vi "ZCR_test_signal_regeneration.vi"() -> ()   [LabVIEW 2020, in "Library Commun.lvlib" / "Nodon_ZCR.lvclass"]
uses:
  Nodon_ZCR.lvclass
  <vilib>/Utility/miscctls.llb/LVRangeTypeDef.ctl
  <vilib>/Analysis/baseanly.llb/Mean (DBL).vi
  <vilib>/measure/matone.llb/Extract Single Tone Information 1 Chan.vi
  Nodon_ZCR.lvclass/Nodon_ZCR.ctl
  <vilib>/measure/NI_MABase.lvlib
  <vilib>/measure/NI_MAPro.lvlib
  <vilib>/Analysis/NI_AALBase.lvlib
  <vilib>/Analysis/NI_AALPro.lvlib
  <vilib>/ptbypt/NI_PtbyPt.lvlib
panel:
  out "FINAL OFF":i32[](array[numeric])
  out "Array 3":i32[](array[numeric])
  out "FINAL ON":i32[](array[numeric])
  out "OFF ARRAY FINAL":i32[](array[numeric])
  out "ON ARRAY FINAL":i32[](array[numeric])
  in  "Coeff":dbl
  in  "Point 2":i32
  out "Delta OFF":i32[](array[numeric])
  out "OFF":i32[](array[numeric])
  out "Array":i32[](array[numeric])
  in  "Point":i32
  out "Waveform Graph 4":waveform(dbl)[](graph)
  out "Waveform Graph 3":waveform(dbl)(graph)
  in  "amplitude":dbl=1.0 format="%.2p"
  out "Waveform Graph 2":waveform(dbl)(graph)
  in  "ZCR ON":waveform(dbl)[](graph)=[{"t0"=timestamp(3707890383.8976955 s since 1904-01-01), "dt"=9.999999999999999e-05, "Y"=array[20000 elements], "attributes"=variant("NI_ChannelName"=variant(string "Tension_0"), "NI_UnitDescription"=variant(string "Volts"))}, {"t0"=timestamp(3707890383.8977456 s since 1904-01-01), "dt"=9.999999999999999e-05, "Y"=array[20000 elements], "attributes"=variant("NI_ChannelName"=variant(string "Tension_1"), "NI_UnitDescription"=variant(string "Volts"))}]
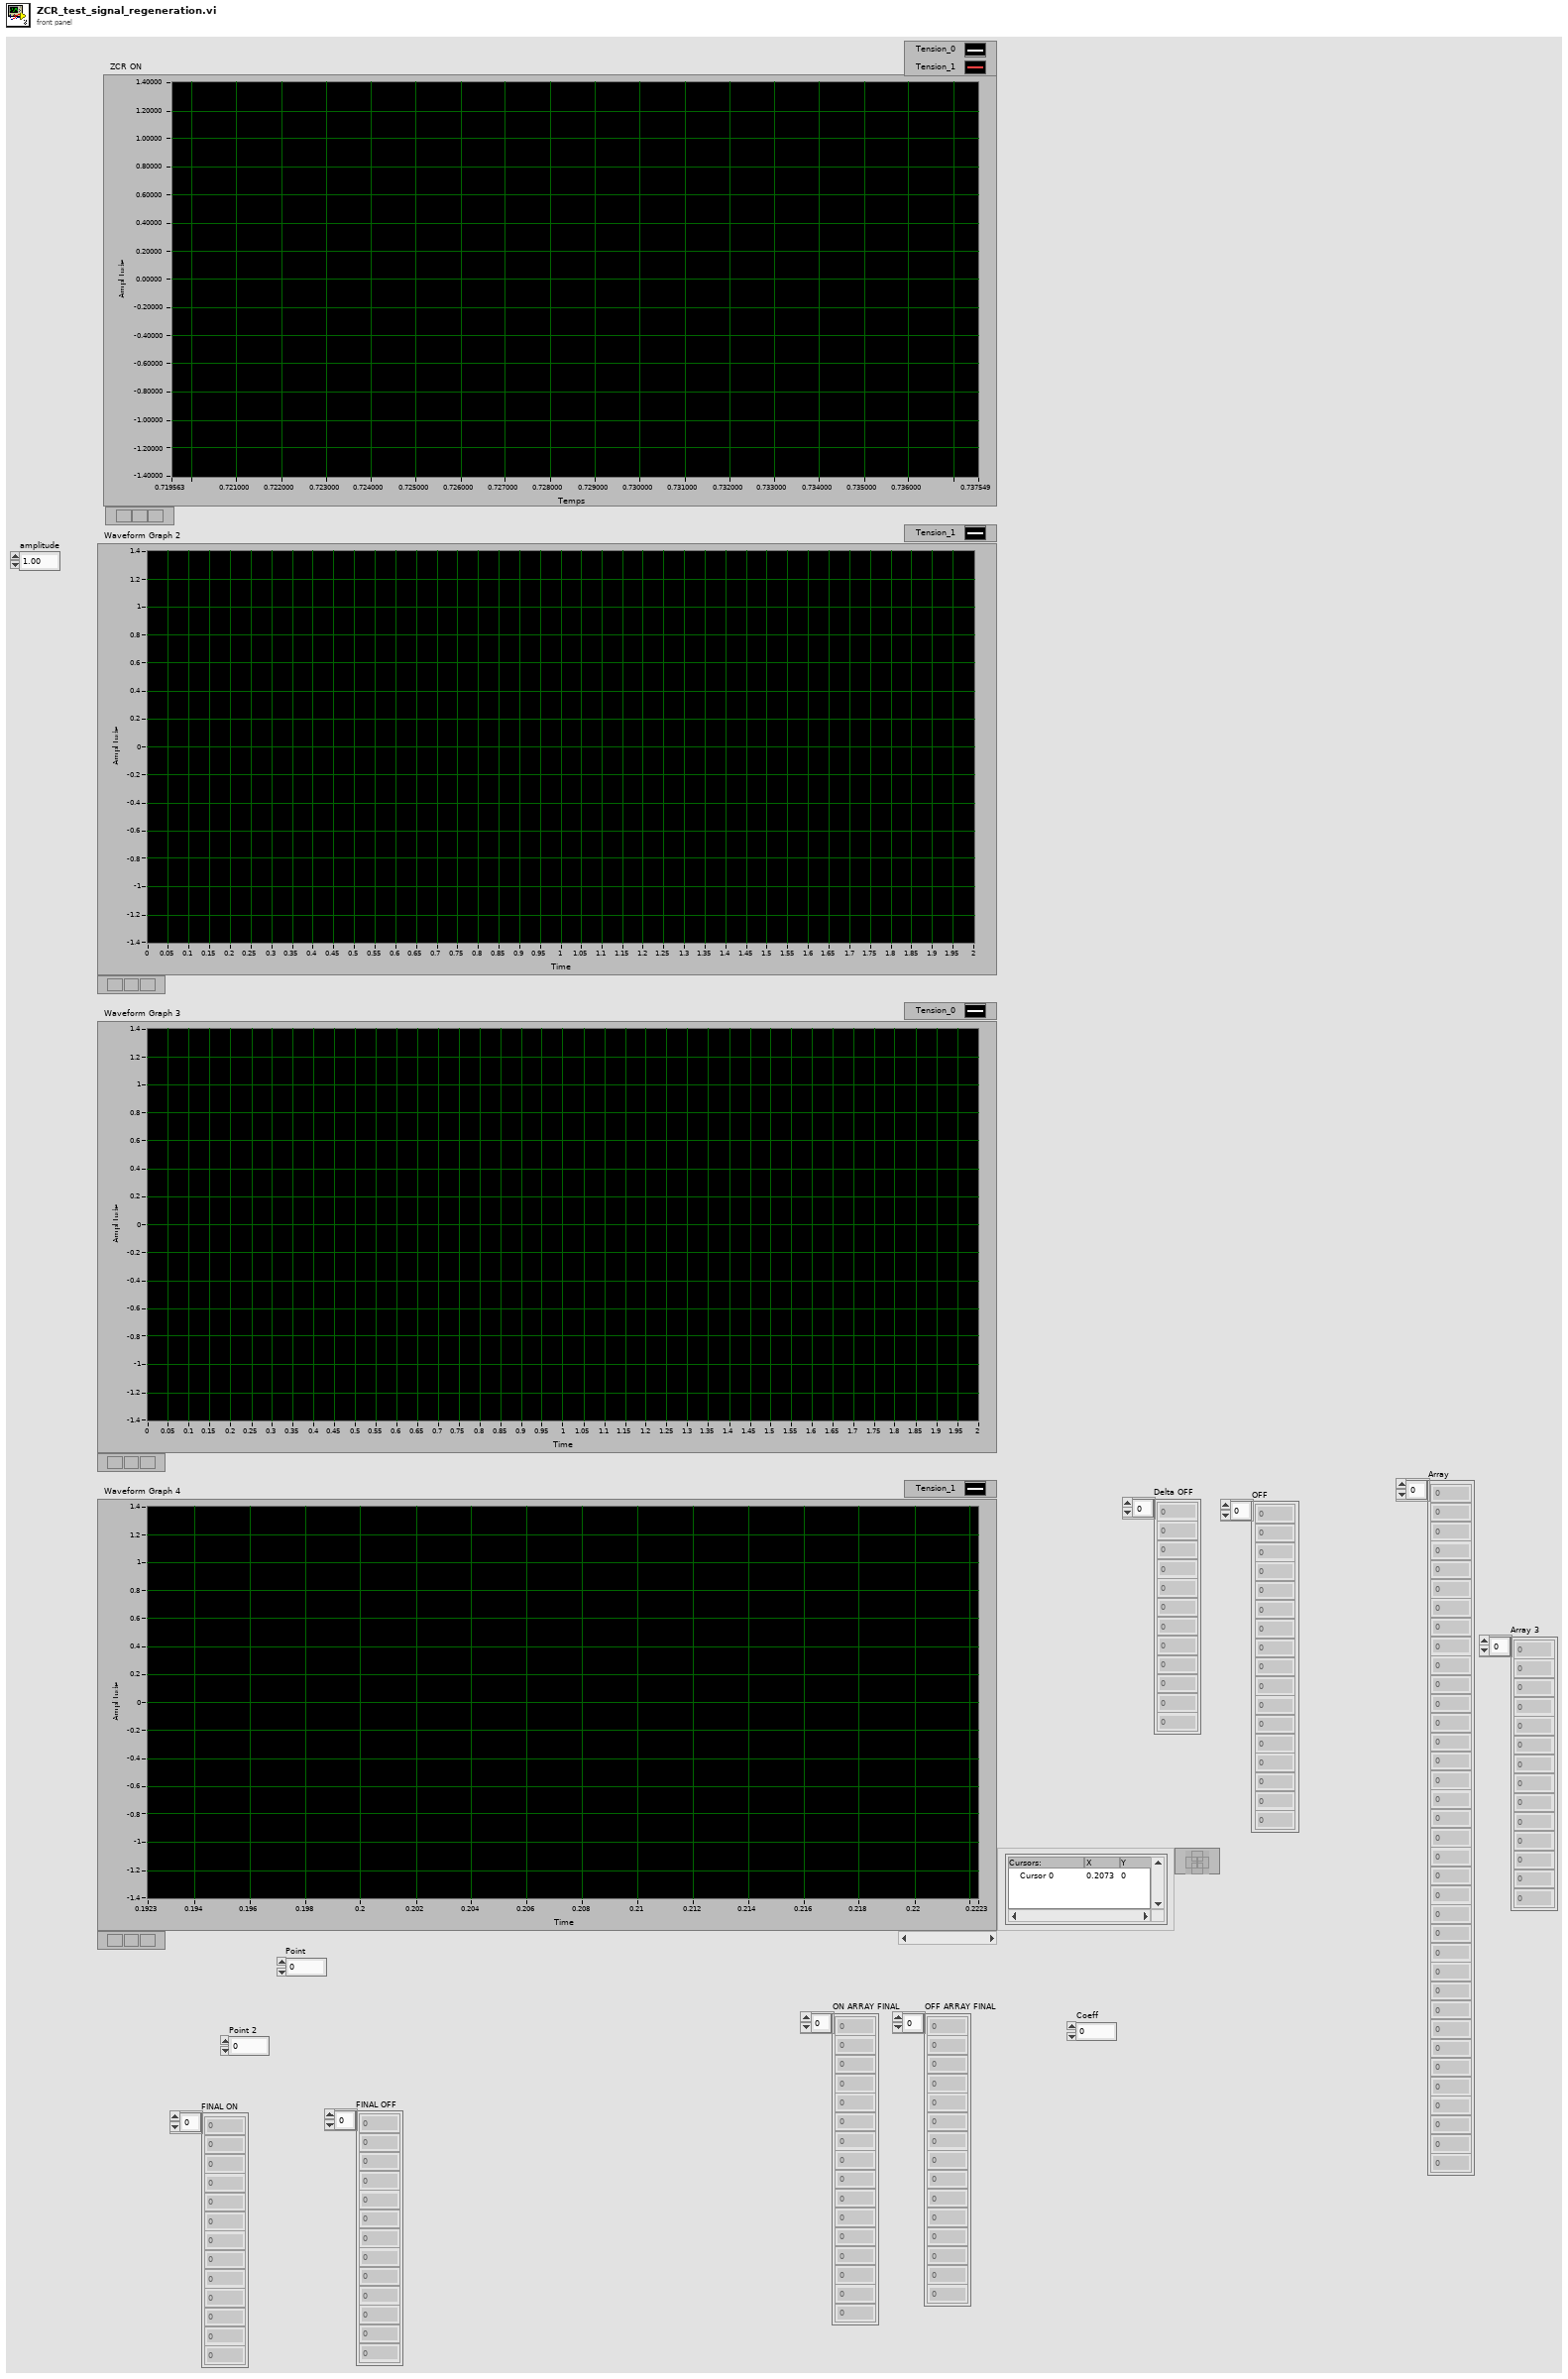
[diagram p1: front panel]
types:
  T1 = typedef "LVRangeTypeDef.ctl" = cluster{"Minimum":dbl, "Maximum":dbl, "Increment":dbl, "Minor Increment":dbl, "Start":dbl}
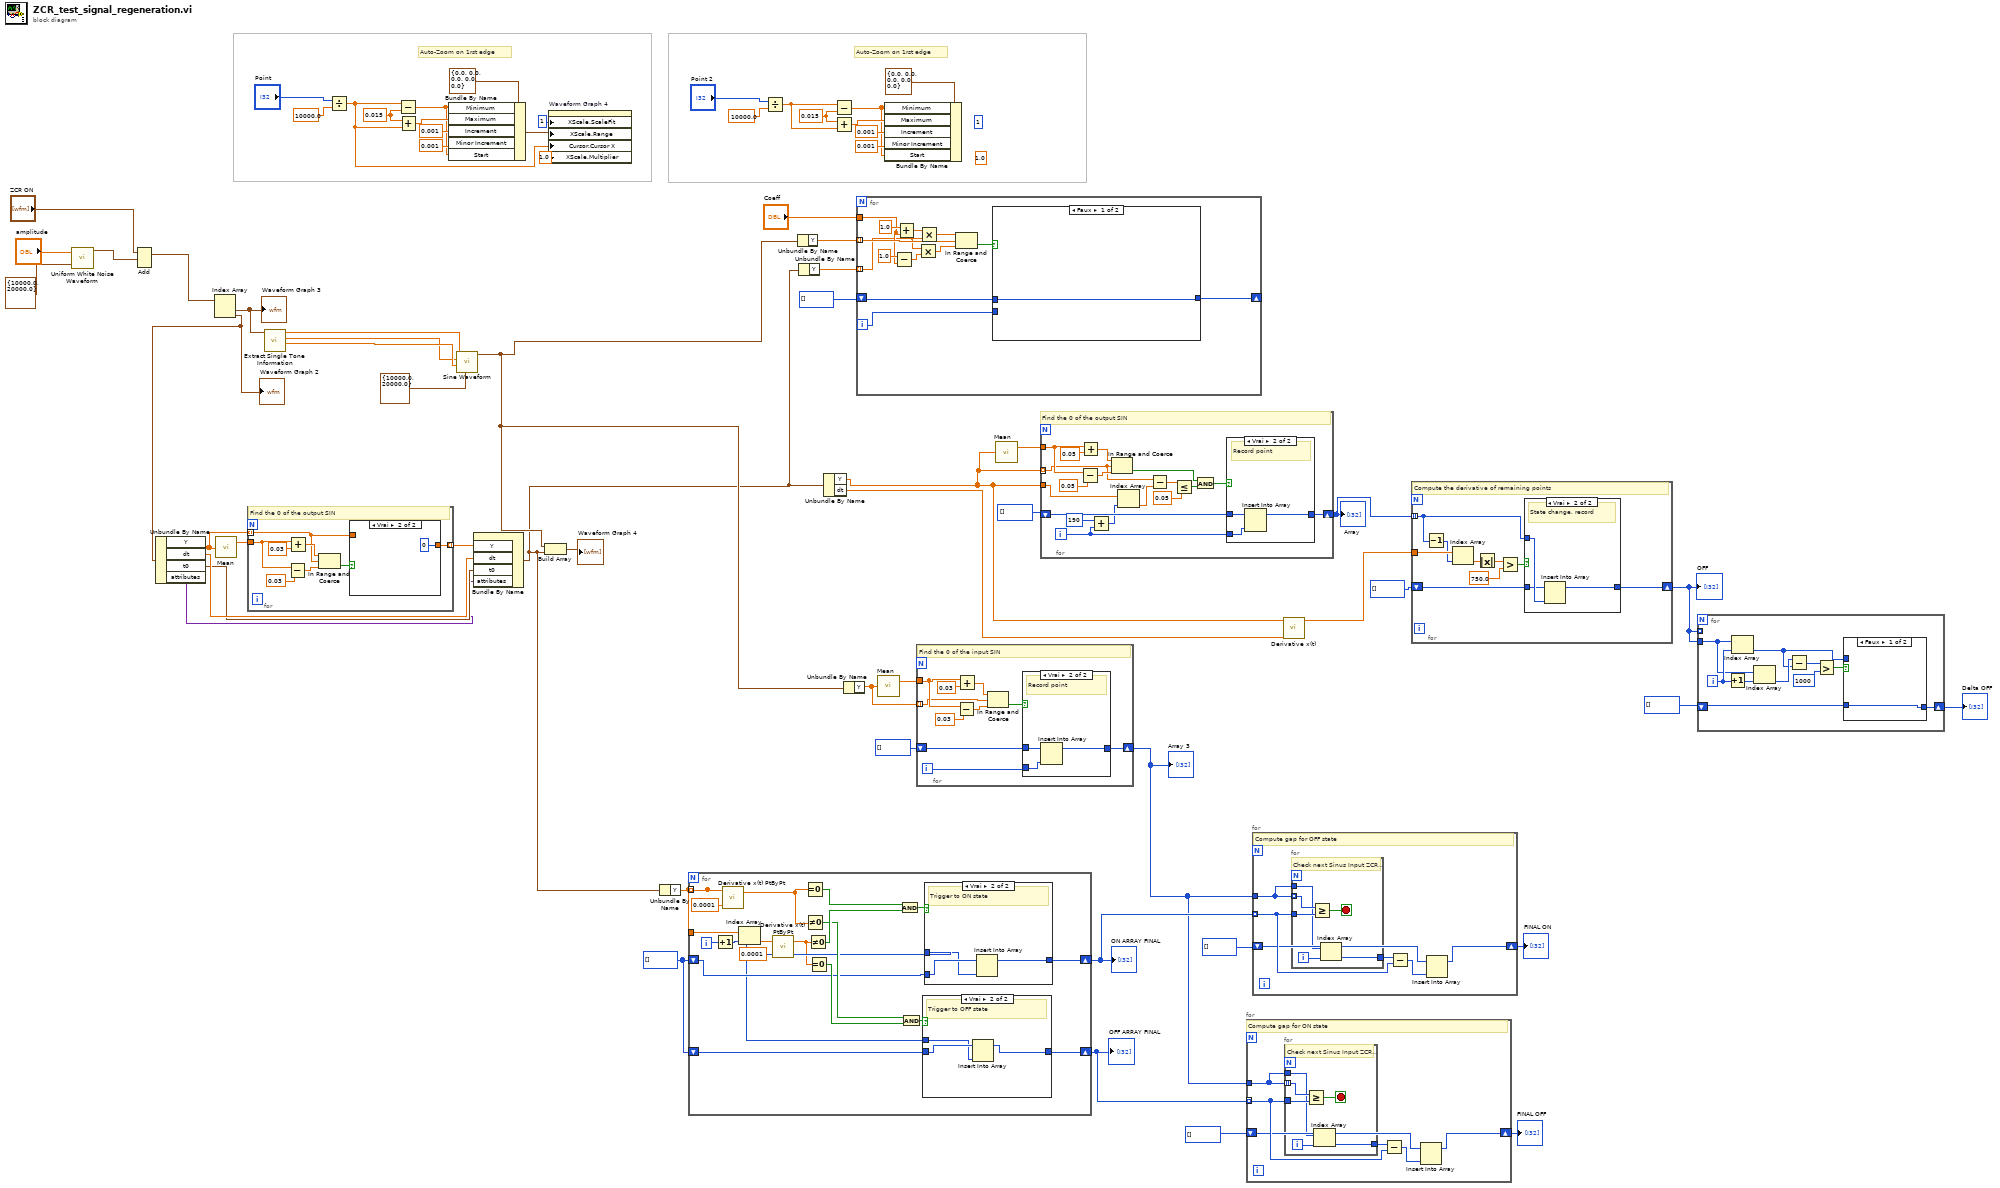
[diagram p0: block diagram]
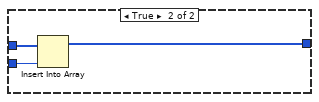
[diagram p5: hidden frame]
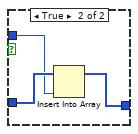
[diagram p7: hidden frame]
diagram:
  w17 = i32[] []
  (unwired) 1.0 ("X Scale.Offset and Multiplier:Multiplier")
  (unwired) u8 1 ("X Scale.Scale Fit")
  w37 = 0.015
  w60 = 0.015
  # "Auto-Zoom on 1rst edge"
  # "Auto-Zoom on 1rst edge"
  n1 = call <vilib>:"Uniform White Noise Waveform.vi"("sampling info"=cluster{"Fs":dbl, "#s":dbl} {"Fs"=10000.0, "#s"=20000.0}, "amplitude"="amplitude") -> ("signal out"=w5:waveform(dbl))  [unwired: 8 in, 1 out]
  n2 = Add(1:w5, 2:"ZCR ON") -> (0:w3:waveform(dbl)[])  [unwired: 1 in, 1 out]
  n3 = Index Array(array=w3) -> (element #1=w21:waveform(dbl), element #2=w4:waveform(dbl))  [unwired: 2 in]
  "Waveform Graph 2" <- w4
  "Waveform Graph 3" <- w21
  n4 = Unbundle By Name(w4) -> ("Y"=w24:dbl[], "dt"=w27:dbl, "t0"=w26:timestamp, "attributes"=w25:variant)
  n5 = call-poly <vilib>:"Mean.vi"("X"=w24) -> ("mean"=w29:dbl)  [unwired: 1 out]
  n6 = for {
    tunnel: w29 -> [w71]
    tunnel: [w69] -> w28 mode=indexing
    tunnel: w24 -> [w68] mode=indexing
    # "Find the 0 of the output SIN"
    n7 = Subtract(x=w71, y=0.03) -> (x-y=w73:dbl)
    n8 = Add(x=w71, y=0.03) -> (x+y=w75:dbl)
    n9 = In Range and Coerce(upper limit=w75, x=w68, lower limit=w73) -> (In Range?=w70:bool)  [unwired: 1 out]
    n10 = case shown="Vrai" w70 {
      tunnel: w68 -> [w76 _]
      tunnel: [w76 0] -> w69
      frame False {
      }
      frame True {
      }
    }
  }
  n11 = call-poly <vilib>:"Extract Single Tone Information.vi"("time signal in"=w21) -> ("detected phase (deg)"=w64:dbl, "detected amplitude"=w63:dbl, "detected frequency"=w62:dbl)  [unwired: 5 in, 3 out]
  n12 = Divide(x="Point", y=10000.0) -> (x/y=w51:dbl)
  n13 = Subtract(x=w51, y=w60) -> (x-y=w55:dbl)
  n14 = Add(x=w60, y=w51) -> (x+y=w58:dbl)
  n15 = Bundle By Name(cluster=T1 {"Minimum"=0.0, "Maximum"=0.0, "Increment"=0.0, "Minor Increment"=0.0, "Start"=0.0} ("X Scale.Range"), "Minimum"=w55, "Maximum"=w58, "Increment"=0.001, "Minor Increment"=0.001, "Start"=w55) -> (w54:T1)
  n16 = call <vilib>:"Sine Waveform.vi"("sampling info"=cluster{"Fs":dbl, "#s":dbl} {"Fs"=10000.0, "#s"=20000.0}, "phase"=w64, "amplitude"=w63, "frequency"=w62) -> ("signal out"=w2:waveform(dbl))  [unwired: 6 in, 1 out]
  n17 = Bundle By Name("Y"=w28, "dt"=w27, "t0"=w26, "attributes"=w25) -> (w1:waveform(dbl))  [unwired: 1 in]
  n18 = Build Array(w2, w1) -> (→"Waveform Graph 4":waveform(dbl)[])
  n19 = property on="Waveform Graph 4" class="GraphWF (strict)"("XScale.ScaleFit"=u8 1 ("X Scale.Scale Fit"), "XScale.Range"=w54, "Cursor.Cursor X"=w51, "XScale.Multiplier"=1.0 ("X Scale.Offset and Multiplier:Multiplier")) -> ()  [unwired: 2 in, 2 out]
  n20 = Unbundle By Name(w1) -> ("Y"=w18:dbl[])
  n21 = for {
    tunnel: [w83] -> _ mode=indexing
    tunnel: w18 -> [w83] mode=indexing
    tunnel: w18 -> [w96]
    shift-right: [w85] -> w11
    shift-left: w17 -> [w88]
    shift-right: [w84] -> w9
    shift-left: w17 -> [w87]
    i -> [w86]
    n22 = Increment(x=w86) -> (x+1=w95:i32)
    n23 = call <vilib>:"Derivative x(t) PtByPt.vi"("dt"=0.0001, "x"=w83) -> ("dx/dt"=w82:dbl)  [unwired: 2 in, 1 out]
    n24 = Index Array(array=w96, index=w95) -> (element=w80:dbl)
    n25 = call <vilib>:"Derivative x(t) PtByPt.vi"("dt"=0.0001, "x"=w80) -> ("dx/dt"=w79:dbl)  [unwired: 2 in, 1 out]
    n26 = Equal To 0?(x=w82) -> (x = 0?=w93:bool)
    n27 = Not Equal To 0?(x=w82) -> (x != 0?=w90:bool)
    n28 = Not Equal To 0?(x=w79) -> (x != 0?=w94:bool)
    n29 = Equal To 0?(x=w79) -> (x = 0?=w91:bool)
    n30 = And(x=w93, y=w94) -> (x .and. y?=w92:bool)
    n31 = And(x=w90, y=w91) -> (x .and. y?=w89:bool)
    n32 = case shown="Vrai" w89 {
      tunnel: w87 -> [w97 w100]
      tunnel: w86 -> [_ w99]
      tunnel: [w97 w98] -> w84
      frame False {
      }
      frame True {
        # "Trigger to OFF state"
        n33 = Insert Into Array(array=w100, new element=w99) -> (w98:i32[])  [unwired: 1 in]
      }
    }
    n34 = case shown="Vrai" w92 {
      tunnel: w88 -> [w101 w104]
      tunnel: w86 -> [_ w103]
      tunnel: [w101 w102] -> w85
      frame False {
      }
      frame True {
        # "Trigger to ON state"
        n35 = Insert Into Array(array=w104, new element=w103) -> (w102:i32[])  [unwired: 1 in]
      }
    }
  }
  "ON ARRAY FINAL" <- w11
  "OFF ARRAY FINAL" <- w9
  n36 = Divide(x="Point 2", y=10000.0) -> (x/y=w31:dbl)
  n37 = Unbundle By Name(w2) -> ("Y"=w23:dbl[])
  n38 = Unbundle By Name(w1) -> ("Y"=w22:dbl[])
  n39 = Unbundle By Name(w1) -> ("Y"=w45:dbl[], "dt"=w44:dbl)
  n40 = Subtract(x=w31, y=w37) -> (x-y=w32:dbl)
  n41 = Add(x=w37, y=w31) -> (x+y=w35:dbl)
  n42 = Unbundle By Name(w2) -> ("Y"=w14:dbl[])
  n43 = for {
    tunnel: w23 -> [w117] mode=indexing
    tunnel: w22 -> [w110] mode=indexing
    tunnel: "Coeff" -> [w114]
    shift-right: [w105] -> _
    shift-left: i32[] [] -> [w107]
    i -> [w106]
    n44 = Subtract(x=1.0, y=w114) -> (x-y=w111:dbl)
    n45 = Add(x=1.0, y=w114) -> (x+y=w113:dbl)
    n46 = Multiply(x=w110, y=w111) -> (x*y=w109:dbl)
    n47 = Multiply(x=w113, y=w110) -> (x*y=w112:dbl)
    n48 = In Range and Coerce(upper limit=w112, x=w117, lower limit=w109) -> (In Range?=w108:bool)  [unwired: 1 out]
    n49 = case shown="Faux" w108 {
      tunnel: w107 -> [w118 w121]
      tunnel: w106 -> [_ w120]
      tunnel: [w118 w119] -> w105
      frame False {
      }
      frame True {
        n50 = Insert Into Array(array=w121, new element=w120) -> (w119:i32[])  [unwired: 1 in]
      }
    }
  }
  n51 = call-poly <vilib>:"Mean.vi"("X"=w14) -> ("mean"=w16:dbl)  [unwired: 1 out]
  n52 = Bundle By Name(cluster=T1 {"Minimum"=0.0, "Maximum"=0.0, "Increment"=0.0, "Minor Increment"=0.0, "Start"=0.0} ("X Scale.Range"), "Minimum"=w32, "Maximum"=w35, "Increment"=0.001, "Minor Increment"=0.001, "Start"=w32) -> ()  [unwired: 1 out]
  n53 = for {
    tunnel: w14 -> [w126] mode=indexing
    tunnel: w16 -> [w127]
    shift-right: [w122] -> w10
    shift-left: i32[] [] -> [w123]
    i -> [w124]
    # "Find the 0 of the input SIN"
    n54 = Subtract(x=w127, y=0.03) -> (x-y=w129:dbl)
    n55 = Add(x=w127, y=0.03) -> (x+y=w131:dbl)
    n56 = In Range and Coerce(upper limit=w131, x=w126, lower limit=w129) -> (In Range?=w125:bool)  [unwired: 1 out]
    n57 = case shown="Vrai" w125 {
      tunnel: w124 -> [_ w135]
      tunnel: w123 -> [w132 w134]
      tunnel: [w132 w133] -> w122
      frame False {
        # "do nothing"
      }
      frame True {
        # "Record point"
        n58 = Insert Into Array(array=w134, new element=w135) -> (w133:i32[])  [unwired: 1 in]
      }
    }
  }
  "Array 3" <- w10
  n59 = call-poly <vilib>:"Mean.vi"("X"=w45) -> ("mean"=w48:dbl)  [unwired: 1 out]
  n60 = for {
    tunnel: w45 -> [w145] mode=indexing
    tunnel: w48 -> [w149]
    shift-right: [w147] -> w46
    shift-left: i32[] [] -> [w148]
    tunnel: w45 -> [w146]
    i -> [w137]
    # "Find the 0 of the output SIN"
    n61 = Subtract(x=w149, y=0.05) -> (x-y=w151:dbl)
    n62 = Add(x=w149, y=0.05) -> (x+y=w153:dbl)
    n63 = Add(x=190, y=w137) -> (x+y=w138:i32)
    n64 = In Range and Coerce(upper limit=w153, x=w145, lower limit=w151) -> (In Range?=w140:bool)  [unwired: 1 out]
    n65 = Index Array(array=w146, index=w138) -> (element=w144:dbl)
    n66 = Subtract(x=w145, y=w144) -> (x-y=w143:dbl)
    n67 = Less Or Equal?(x=w143, y=0.05) -> (x <= y?=w141:bool)
    n68 = And(x=w140, y=w141) -> (x .and. y?=w139:bool)
    n69 = case shown="Vrai" w139 {
      tunnel: w137 -> [_ w157]
      tunnel: w148 -> [w154 w156]
      tunnel: [w154 w155] -> w147
      frame False {
        # "do nothing"
      }
      frame True {
        # "Record point"
        n70 = Insert Into Array(array=w156, new element=w157) -> (w155:i32[])  [unwired: 1 in]
      }
    }
  }
  "Array" <- w46
  n71 = for {
    tunnel: w9 -> [w161] mode=indexing
    tunnel: w10 -> [w163]
    shift-right: [w158] -> w7
    shift-left: i32[] [] -> [w160]
    # "Compute gap for ON state"
    n72 = for {
      tunnel: w163 -> [w169] mode=indexing
      tunnel: w161 -> [w168]
      tunnel: w163 -> [w166]
      tunnel: [w165] -> w162
      i -> [w164]
      stop <- w167 stop-if-true
      # "Check next Sinus Input ZCR crossing"
      n73 = Greater Or Equal?(x=w169, y=w168) -> (x >= y?=w167:bool)
      n74 = Index Array(array=w166, index=w164) -> (element=w165:i32)
    }
    n75 = Subtract(x=w162, y=w161) -> (x-y=w159:i32)
    n76 = Insert Into Array(array=w160, new element=w159) -> (w158:i32[])  [unwired: 1 in]
  }
  "FINAL OFF" <- w7
  n77 = for {
    tunnel: w11 -> [w173] mode=indexing
    tunnel: w10 -> [w175]
    shift-right: [w170] -> w13
    shift-left: i32[] [] -> [w172]
    # "Compute gap for OFF state"
    n78 = for {
      tunnel: w175 -> [w181] mode=indexing
      tunnel: w173 -> [w180]
      tunnel: w175 -> [w178]
      tunnel: [w177] -> w174
      i -> [w176]
      stop <- w179 stop-if-true
      # "Check next Sinus Input ZCR crossing"
      n79 = Greater Or Equal?(x=w181, y=w180) -> (x >= y?=w179:bool)
      n80 = Index Array(array=w178, index=w176) -> (element=w177:i32)
    }
    n81 = Subtract(x=w174, y=w173) -> (x-y=w171:i32)
    n82 = Insert Into Array(array=w172, new element=w171) -> (w170:i32[])  [unwired: 1 in]
  }
  "FINAL ON" <- w13
  n83 = call <vilib>:"Derivative x(t).vi"("dt"=w44, "X"=w45) -> ("dX/dt"=w43:dbl[])  [unwired: 8 in, 1 out]
  n84 = for {
    tunnel: w46 -> [w182] mode=indexing
    shift-right: [w189] -> w41
    shift-left: i32[] [] -> [w190]
    tunnel: w43 -> [w188]
    # "Compute the derivative of remaining points"
    n85 = Decrement(x=w182) -> (x-1=w183:i32)
    n86 = Index Array(array=w188, index=w183) -> (element=w187:dbl)
    n87 = Absolute Value(x=w187) -> (abs(x)=w186:dbl)
    n88 = Greater?(x=w186, y=750.0) -> (0:w184:bool)
    n89 = case shown="Vrai" w184 {
      tunnel: w190 -> [w191 w192]
      tunnel: [w191 w193] -> w189
      tunnel: w182 -> [_ w194]
      frame False {
        # "Same state as N-1 (0), do nothing"
      }
      frame True {
        # "State change, record"
        n90 = Insert Into Array(array=w192, new element=w194) -> (w193:i32[])  [unwired: 1 in]
      }
    }
  }
  "OFF" <- w41
  n91 = for {
    tunnel: w41 -> [w196]
    tunnel: w41 -> [_] mode=indexing
    shift-right: [w197] -> w39
    shift-left: i32[] [] -> [w198]
    i -> [w203]
    n92 = Increment(x=w203) -> (x+1=w204:i32)
    n93 = Index Array(array=w196, index=w203) -> (element=w195:i32)
    n94 = Index Array(array=w196, index=w204) -> (element=w202:i32)
    n95 = Subtract(x=w202, y=w195) -> (x-y=w201:i32)
    n96 = Greater?(x=w201, y=1000) -> (0:w199:bool)
    n97 = case shown="Faux" w199 {
      tunnel: w198 -> [w205 w208]
      tunnel: [w205 w207] -> w197
      tunnel: w195 -> [_ w206]
      frame False {
      }
      frame True {
        n98 = Insert Into Array(array=w208, new element=w206) -> (w207:i32[])  [unwired: 1 in]
      }
    }
  }
  "Delta OFF" <- w39
